vi "Print Debug String.vi"(7 "error in":errorcluster, 9 "Color (Plain White)":u16(ring)=7 items=["Plain White"=7, "Bold White"=15, "Bold Blue"=9, "Bold Green"=10, "Bold Red"=12], 10 "String to write":string) -> (0 "error out":errorcluster)   [LabVIEW 2019, in "SEECD Engine.lvlib"]
doc: "Prints error information out to the console. Provide your code's public name. For example, if your code is about J1939, put that here so the user knows what this printed error information has to do with.\n\nIf this is not a NI VeriStand custom device, write false to the Custom Device? input. This will change the error output and cause this to ignore error -2206.\n\nIf the 'note' field is empty, it is not printed to the console.\n\nExample output 1:\n******J1939 ERROR******\nSource: blah.vi\nCode: 535\n******J1939 ERROR******\n\nExample output 2:\n******XCP and CCP Master CUSTOM DEVICE ERROR******\nSource: blah.vi\nCode: 535\nUser Note: before write\n******XCP and CCP Master CUSTOM DEVICE ERROR******"
uses:
  SEECD Engine.lvlib
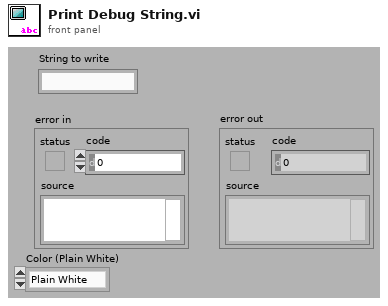
[diagram p1: front panel]
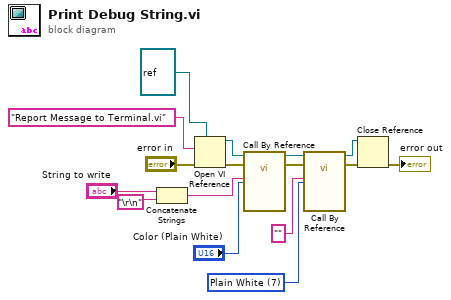
[diagram p0: block diagram]
diagram:
  w11 = u16 7 items=["Plain White"=7, "Bold White"=15, "Bold Blue"=9, "Bold Green"=10, "Bold Red"=12] ("Color (Plain White)")
  n1 = Concatenate Strings("String to write", "\r\n") -> (w10:string)
  n2 = Open VI Reference(type specifier VI Refnum (for type only)=refnum<vi> refnum, vi path="Report Message to Terminal.vi", error in (no error)="error in") -> (vi reference=w9:refnum<vi>, error out=w8:errorcluster)  [unwired: 1 in, 2 out]
  n3 = call-by-ref "?"(reference=w9, error in=w8, "Color (Plain White)"="Color (Plain White)", "Message"=w10) -> (reference out=w4:refnum<vi>, error out=w3:errorcluster)  [unwired: 9 in, 1 out]
  n4 = call-by-ref "?"(reference=w4, error in=w3, "Color (Plain White)"=w11, "Message"="") -> (reference out=w12:refnum<vi>, error out=w13:errorcluster)  [unwired: 9 in, 1 out]
  n5 = Close Reference(reference=w12, error in (no error)=w13) -> (error out=→"error out":errorcluster)
